vi "OpenBLAS_RT_Set_Threads.vi"(8 "error in (no error)":errorcluster, 11 "threads":i32=3) -> (0 "error out":errorcluster)   [LabVIEW 2024]
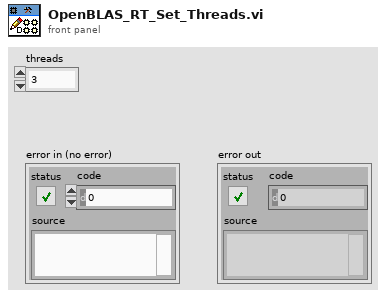
[diagram p1: front panel]
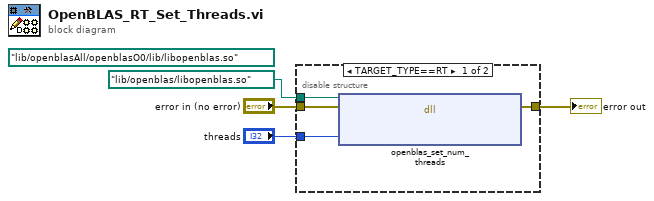
[diagram p0: block diagram]
diagram:
  (unwired) path "/lib/openblasAll/openblasO0/lib/libopenblas.so" ("path in")
  n1 = disable-structure shown="TARGET_TYPE==RT" {
    disable-tunnel: "threads" -> [w8 _]
    disable-tunnel: [w7 w9] -> w3
    disable-tunnel: path "/lib/openblas/libopenblas.so" ("path in") -> [w6 _]
    disable-tunnel: "error in (no error)" -> [w5 w9]
    frame condition #0 (active) {
      n2 = dll-call lib="?" fn="openblas_set_num_threads" ("CBLAS.dll:MtrxxVectH")(path in=w6, error in=w5, "threads"=w8) -> (error out=w7:errorcluster)  [unwired: 1 in, 3 out]
    }
    frame condition #1 {
    }
  }
  "error out" <- w3
